vi "direction_axis.vi"(9 "Direction":T1, 10 "backwardaxis":i16, 11 "forwardaxis":i16) -> (1 "Slave":i16, 3 "Master":i16)   [LabVIEW 2013, in "Tapedrive_ESP301.lvclass"]
uses:
  Tapedrive_ESP301.lvclass
  Direction.ctl
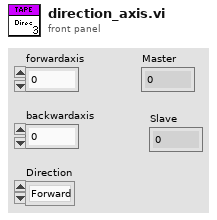
[diagram p1: front panel]
types:
  T1 = typedef "Direction.ctl" = enum16{"Forward", "Backward", "Undefined"}
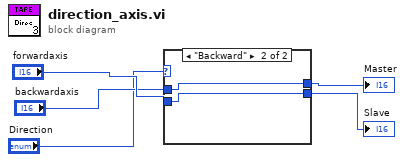
[diagram p0: block diagram]
diagram:
  n1 = case shown="\"Backward\"" "Direction" {
    tunnel: [w7 w9] -> w5
    tunnel: "backwardaxis" -> [w6 w9]
    tunnel: "forwardaxis" -> [w7 w8]
    tunnel: [w6 w8] -> w1
    frame "Forward", Default {
    }
    frame "Backward" {
    }
  }
  "Master" <- w5
  "Slave" <- w1
